vi "Get Data For Report.vi"(8 "error constant":errorcluster, 11 "Channel Tags":string[](array[string])) -> (0 "error out":errorcluster, 3 "Value":dbl[](array[numeric]))   [LabVIEW 2018]
uses:
  Globals/Host Globals.vi
  <vilib>/Utility/error.llb/Error Cluster From Error Code.vi
  <vilib>/ErrorRing/Error Ring.xnode
  Modules/Controller (Host)/Controller (Host).lvlib
panel:
  out "Error Out":errorcluster
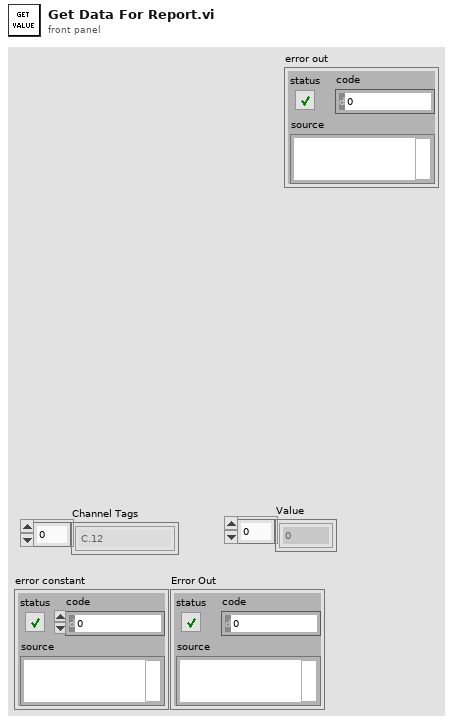
[diagram p1: front panel]
types:
  T1 = typedef "Calculated Data.ctl" = cluster{"C.00":dbl, "C.01":dbl, "C.02":dbl, "C.03":dbl, "C.04":dbl, "C.05":dbl, "C.06":dbl, "C.07":dbl, "C.08":dbl, "C.09":dbl, "C.10":dbl, "C.11":dbl, "C.12":dbl, "C.13":dbl, "C.14":dbl, "C.15":dbl, "C.16":dbl, "C.17":dbl, "C.18":dbl, "C.19":dbl, "C.20":dbl, "C.21":dbl, "C.22":dbl, "C.23":dbl, "C.24":dbl, "C.25":dbl, "C.26":dbl, "C.27":dbl, "C.28":dbl, "C.29":dbl, "C.30":dbl, "C.31":dbl, "C.32":dbl, "C.33":dbl, "C.34":dbl, "C.35":dbl, "C.36":dbl, "C.37":dbl, "C.38":dbl, "C.39":dbl, "C.40":dbl, "C.41":dbl, "C.42":dbl, "C.43":dbl, "C.44":dbl, "C.45":dbl, "C.46":dbl, "C.47":dbl, "C.48":dbl, "C.49":dbl, "C.50":dbl, "C.51":dbl, "C.52":dbl, "C.53":dbl, "C.54":dbl, "C.55":dbl, "C.56":dbl, "C.57":dbl, "C.58":dbl, "C.59":dbl, "C.60":dbl, "C.61":dbl, "C.62":dbl}
  T2 = typedef "All Data Cluster.ctl" = cluster{"AI":T3, "Accel Data":cluster{"Accel RMS(in/sec2)":dbl[], "Accel Peak(in/sec2)":dbl[], "Velocity RMS(in/sec)":dbl[], "Velocity Peak(in/sec)":dbl[]}, "Temps":cluster{"01-00-9213":dbl[], "01-01-9213":dbl[], "01-02-9213":dbl[]}, "00-03-9402(RPM)":dbl[], "02-04-9871":dbl[], "ARINC":sgl[]}
  T3 = typedef "Acq Data.ctl" = cluster{"00-00-9220":dbl[], "00-01-9220":dbl[], "02-02-9219":dbl[], "02-03-9227":dbl[], "02-05-9205":dbl[]}
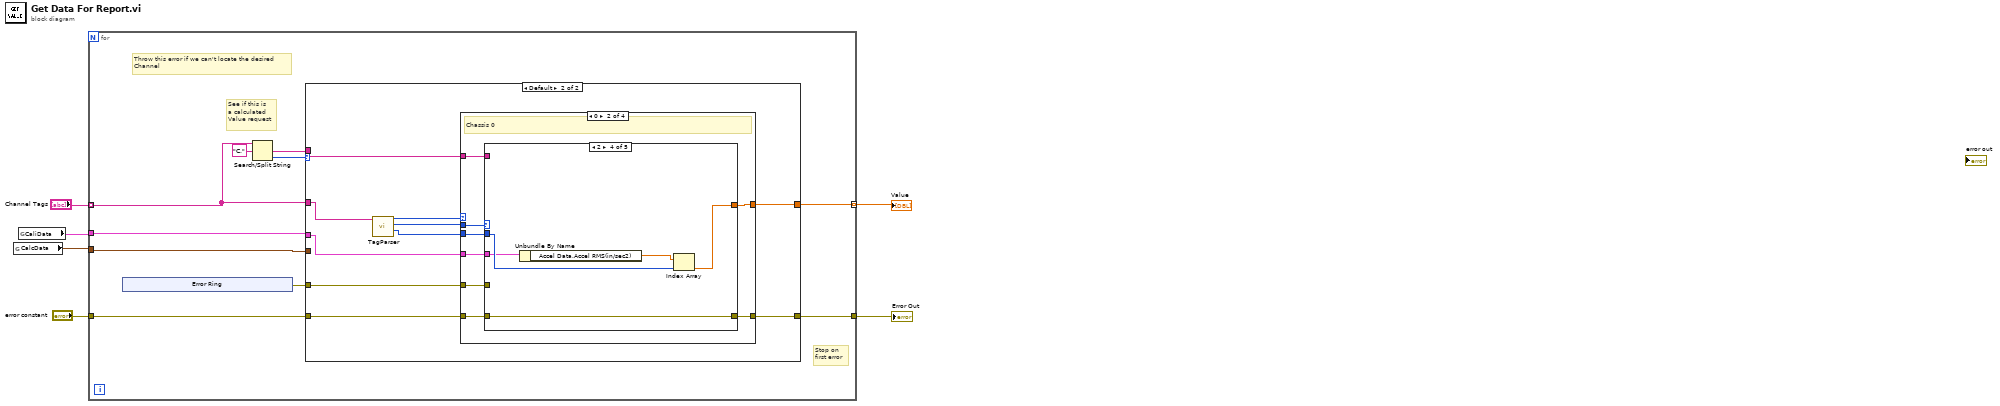
[diagram p0: block diagram]
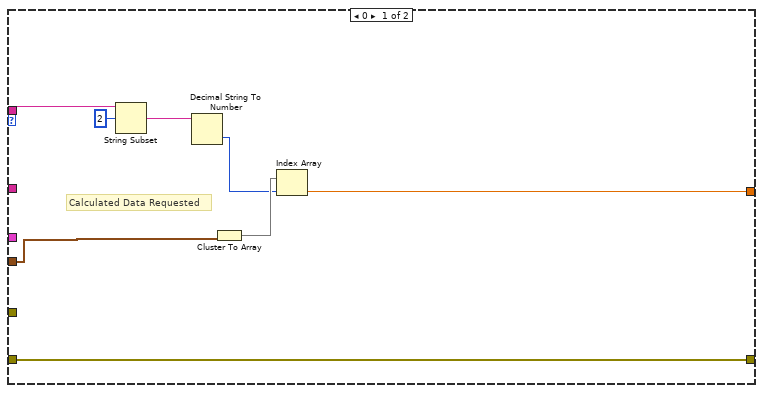
[diagram p2: hidden frame]
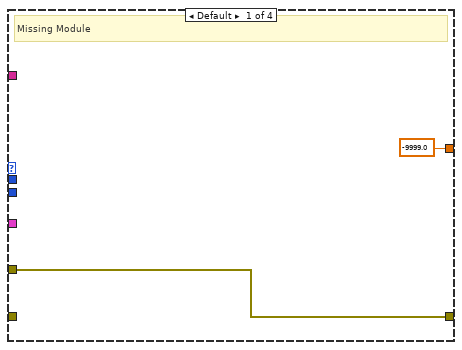
[diagram p3: hidden frame]
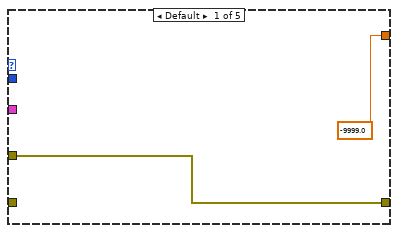
[diagram p4: hidden frame]
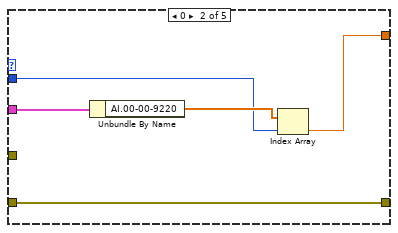
[diagram p5: hidden frame]
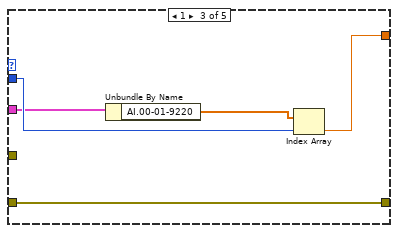
[diagram p6: hidden frame]
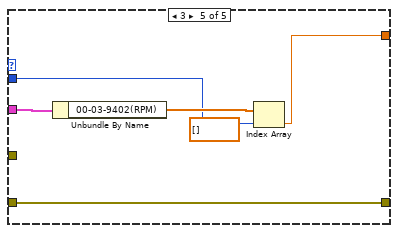
[diagram p7: hidden frame]
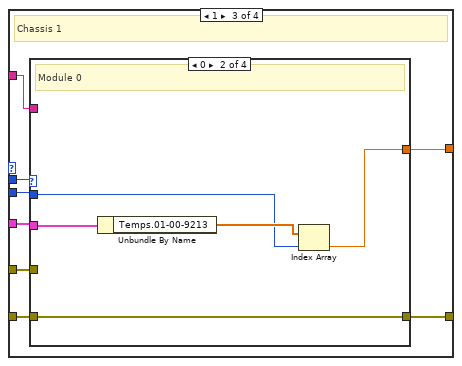
[diagram p8: hidden frame]
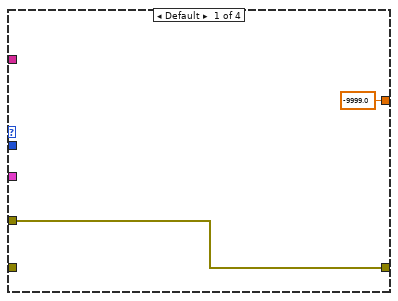
[diagram p9: hidden frame]
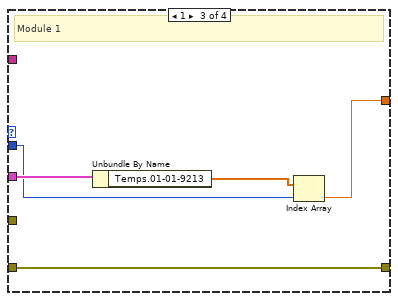
[diagram p10: hidden frame]
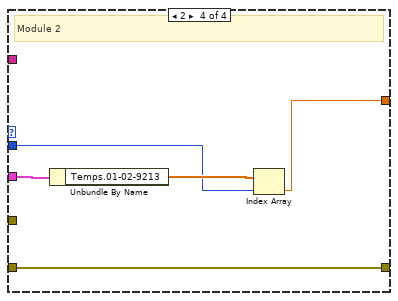
[diagram p11: hidden frame]
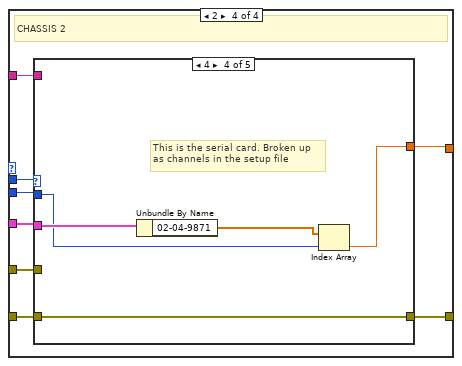
[diagram p12: hidden frame]
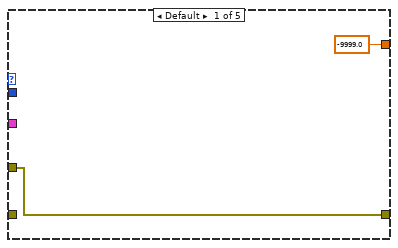
[diagram p13: hidden frame]
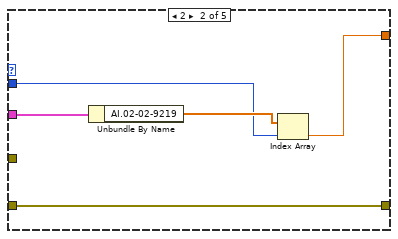
[diagram p14: hidden frame]
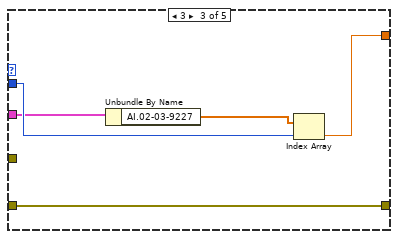
[diagram p15: hidden frame]
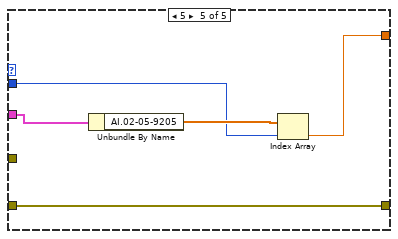
[diagram p16: hidden frame]
diagram:
  n1 = global read "Host Globals.vi" "CalcData"() -> (w2:T1)
  n2 = global read "Host Globals.vi" "CaliData"() -> (w1:T2)
  n3 = for {
    tunnel: "Channel Tags" -> [w15] mode=indexing
    tunnel: [w10] -> w3 mode=indexing
    tunnel: "error constant" -> [w16]
    tunnel: [w9] -> w6
    tunnel: w1 -> [w8]
    tunnel: w2 -> [w7]
    # "Stop on\nfirst error"
    # "See if this is\na calculated\nValue request"
    # "Throw this error if we can't locate the desired\nChannel"
    n4 = xnode "Error Ring"() -> ("error out"=w11:errorcluster)
    n5 = Search/Split String(string=w15, search string/char (-)="C.") -> (match + rest of string=w12:string, offset of match=w13:i32)  [unwired: 1 in, 1 out]
    n6 = case shown="Default" w13 {
      tunnel: w15 -> [_ w33]
      tunnel: w12 -> [w29 w34]
      tunnel: [w24 w39] -> w10
      tunnel: w8 -> [_ w38]
      tunnel: w16 -> [w23 w37]
      tunnel: w11 -> [_ w36]
      tunnel: [w23 w35] -> w9
      tunnel: w7 -> [w22 _]
      frame 0 {
        # "Calculated Data Requested"
        n7 = String Subset(string=w29, offset (0)=2) -> (substring=w27:string)  [unwired: 1 in]
        n8 = Decimal String To Number(string=w27) -> (number=w25:i32)  [unwired: 2 in, 1 out]
        n9 = Cluster To Array(cluster=w22) -> (array=w26:dbl[])
        n10 = Index Array(array=w26, index=w25) -> (element=w24:dbl)
      }
      frame Default {
        n11 = call "TagParser.vi"("Channel Tag"=w33) -> ("Channel"=w30:i32, "Module"=w31:i32, "Chassis"=w32:i32)  [unwired: 8 in]
        n12 = case shown="0" w32 {
          tunnel: w31 -> [_ w49 w77 w103]
          tunnel: w38 -> [_ w48 w79 w102]
          tunnel: w30 -> [_ w47 w78 w104]
          tunnel: [-9999.0 ("Numeric") w46 w76 w100] -> w39
          tunnel: w34 -> [_ w45 w75 w101]
          tunnel: w37 -> [_ w44 w72 w99]
          tunnel: w36 -> [w40 w43 w74 w97]
          tunnel: [w40 w42 w73 w98] -> w35
          frame Default {
            # "Missing Module"
          }
          frame 0 {
            # "Chassis 0"
            n13 = case shown="2" w49 {
              tunnel: w48 -> [_ w52 w57 w62 w71]
              tunnel: w47 -> [_ w55 w60 w65 w69]
              tunnel: [-9999.0 ("Numeric") w54 w59 w64 w68] -> w46
              tunnel: w45 -> [_ _ _ _ _]
              tunnel: w44 -> [_ w53 w58 w63 w67]
              tunnel: w43 -> [w50 _ _ _ _]
              tunnel: [w50 w53 w58 w63 w67] -> w42
              frame Default {
              }
              frame 0 {
                n14 = Unbundle By Name(w52) -> ("AI.00-00-9220"=w56:dbl[])
                n15 = Index Array(array=w56, index=w55) -> (element=w54:dbl)
              }
              frame 1 {
                n16 = Unbundle By Name(w57) -> ("AI.00-01-9220"=w61:dbl[])
                n17 = Index Array(array=w61, index=w60) -> (element=w59:dbl)
              }
              frame 2 {
                n18 = Unbundle By Name(w62) -> ("Accel Data.Accel RMS(in/sec2)"=w66:dbl[])
                n19 = Index Array(array=w66, index=w65) -> (element=w64:dbl)
              }
              frame 3 {
                (unwired) dbl[] [] ("00-03-9402")
                n20 = Unbundle By Name(w71) -> ("00-03-9402(RPM)"=w70:dbl[])
                n21 = Index Array(array=w70, index=w69) -> (element=w68:dbl)
              }
            }
          }
          frame 1 {
            # "Chassis 1"
            n22 = case shown="0" w77 {
              tunnel: w79 -> [_ w86 w91 w96]
              tunnel: w78 -> [_ w84 w89 w94]
              tunnel: [-9999.0 ("Numeric") w83 w88 w93] -> w76
              tunnel: w75 -> [_ _ _ _]
              tunnel: w74 -> [w80 _ _ _]
              tunnel: [w80 w82 w87 w92] -> w73
              tunnel: w72 -> [_ w82 w87 w92]
              frame Default {
              }
              frame 0 {
                # "Module 0"
                n23 = Unbundle By Name(w86) -> ("Temps.01-00-9213"=w85:dbl[])
                n24 = Index Array(array=w85, index=w84) -> (element=w83:dbl)
              }
              frame 1 {
                # "Module 1"
                n25 = Unbundle By Name(w91) -> ("Temps.01-01-9213"=w90:dbl[])
                n26 = Index Array(array=w90, index=w89) -> (element=w88:dbl)
              }
              frame 2 {
                # "Module 2"
                n27 = Unbundle By Name(w96) -> ("Temps.01-02-9213"=w95:dbl[])
                n28 = Index Array(array=w95, index=w94) -> (element=w93:dbl)
              }
            }
          }
          frame 2 {
            # "CHASSIS 2"
            n29 = case shown="4" w103 {
              tunnel: w102 -> [_ w111 w112 w121 w122]
              tunnel: w104 -> [_ w109 w115 w117 w125]
              tunnel: [-9999.0 ("Numeric") w108 w114 w119 w124] -> w100
              tunnel: w101 -> [_ _ _ _ _]
              tunnel: w99 -> [_ w107 w113 w118 w123]
              tunnel: [w105 w107 w113 w118 w123] -> w98
              tunnel: w97 -> [w105 _ _ _ _]
              frame Default {
              }
              frame 2 {
                n30 = Unbundle By Name(w111) -> ("AI.02-02-9219"=w110:dbl[])
                n31 = Index Array(array=w110, index=w109) -> (element=w108:dbl)
              }
              frame 3 {
                n32 = Unbundle By Name(w112) -> ("AI.02-03-9227"=w116:dbl[])
                n33 = Index Array(array=w116, index=w115) -> (element=w114:dbl)
              }
              frame 4 {
                # "This is the serial card. Broken up \nas channels in the setup file"
                n34 = Unbundle By Name(w121) -> ("02-04-9871"=w120:dbl[])
                n35 = Index Array(array=w120, index=w117) -> (element=w119:dbl)
              }
              frame 5 {
                n36 = Unbundle By Name(w122) -> ("AI.02-05-9205"=w126:dbl[])
                n37 = Index Array(array=w126, index=w125) -> (element=w124:dbl)
              }
            }
          }
        }
      }
    }
  }
  "Error Out" <- w6
  "Value" <- w3
